vi "Get IDs or Error.vi"(0 "RegisteredHandler MsgPack in":refnum<class "RegisteredHandler MsgPack.lvclass">, 11 "error in (no error)":errorcluster) -> (4 "RegisteredHandler MsgPack out":refnum<class "RegisteredHandler MsgPack.lvclass">, 6 "Request ID":u64, 8 "Registration ID":u64, 10 "ErrorOrSuccess":refnum<class "ErrorOrSuccess.lvclass">, 15 "error out":errorcluster)   [LabVIEW 2020, in "wamplv.lvlib" / "RegisteredHandler MsgPack.lvclass"]
uses:
  RegisteredHandler MsgPack.lvclass
  RegisteredHandler MsgPack.lvclass/RegisteredHandler MsgPack.ctl
  Message loop classes/ErrorOrSuccess/ErrorOrSuccess.lvclass
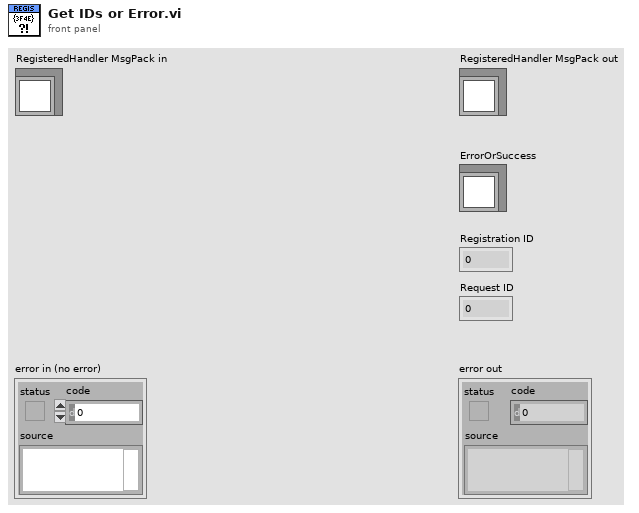
[diagram p1: front panel]
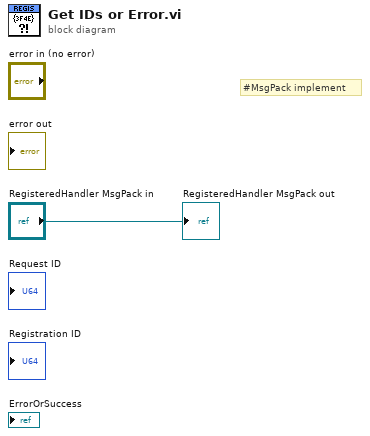
[diagram p0: block diagram]
diagram:
  # "#MsgPack implement"
  "RegisteredHandler MsgPack out" <- "RegisteredHandler MsgPack in"
